vi "Do Wrapper.vi"(8 "error in (no error)":errorcluster, 11 "Actor in":refnum<class "Actor.lvclass">) -> (0 "error out":errorcluster, 3 "Controller out":refnum<class "Controller.lvclass">)   [LabVIEW 2014, in "Controller.lvlib" / "Start Tau Write MSG.lvclass"]
uses:
  Start Tau Write MSG.lvclass
  Controller.lvclass
  File Actor/File Actor.lvclass
  Execute Write Taus/Exe Write Taus.lvclass
  <vilib>/ActorFramework/Actor/Actor.lvclass
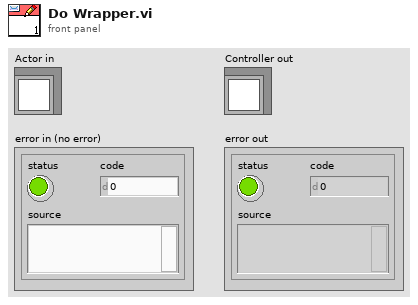
[diagram p1: front panel]
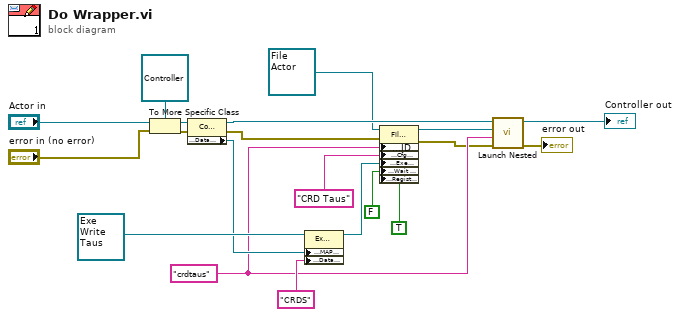
[diagram p0: block diagram]
diagram:
  w5 = "crdtaus" ("ID")
  n1 = To More Specific Class(target class=refnum<class "Controller.lvclass"> refnum ("Controller:Controller"), reference="Actor in", error in="error in (no error)") -> (specific class reference=w7:refnum<class "Controller.lvclass">, error out=w8:errorcluster)
  n2 = property class="Controller"(reference=w7, error in=w8) -> (reference out=w9:refnum<class "Controller.lvclass">, error out=w10:errorcluster, "Accessors:Data Map"=w11:refnum<data-value>)
  n3 = property class="Exe Write Taus"(reference=refnum<class "Exe Write Taus.lvclass"> refnum ("Controller:Exe Write Taus"), "Accessors:MAP DVR"=w11, "Accessors:DataObj"="CRDS" ("DataObj")) -> (reference out=w12:refnum<class "Exe Write Taus.lvclass">)  [unwired: 1 in, 1 out]
  n4 = property class="File Actor"(reference=refnum<class "File Actor.lvclass"> refnum ("File Library.lvlib:File Actor"), error in=w10, "Accessors:ID"=w5, "Accessors:Cfg Header"="CRD Taus" ("Cfg Header"), "Accessors:Exe Write"=w12, "Accessors:Wait on Registration_"=FALSE ("Wait on Registration_"), "Accessors:Registration Complete"=TRUE ("Registration Complete")) -> (reference out=w2:refnum<class "File Actor.lvclass">, error out=w3:errorcluster)
  n5 = call "Launch Nested.vi"("Error In"=w3, "ID"=w5, "Nested Actor"=w2, "Controller in"=w9) -> ("Error Out"=→"error out":errorcluster, "Controller out"=→"Controller out":refnum<class "Controller.lvclass">)  [unwired: 5 in, 1 out]
